vi "PH_ImageOperator.Fill Factor.vi"(0 "i ref in":refnum<vi>, 5 "error in":errorcluster) -> (14 "i ref out":refnum<vi>, 19 "error out":errorcluster)   [LabVIEW 2014, in "PH_ImageOperator.lvlib"]
doc: "This VI calculates the Fill factor."
uses:
  PH_ImageOperator.lvlib
  <vilib>/vision/NI_Vision_Development_Module.lvlib
  PH_Basics/PH_Common/PH_Common.lvlib
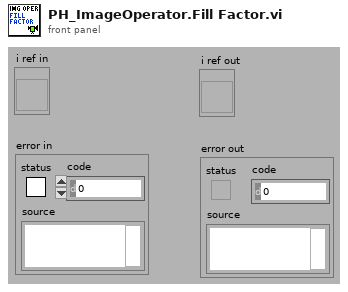
[diagram p1: front panel]
types:
  T1 = typedef "PH_ImageOperator.lvlib/PH_ImageOperator.i attribute.ctl" = cluster{"GUI Refs":cluster{"Delete":refnum<vi>, "Calibration status":refnum<vi>, "BI subtracted":refnum<vi>, "calc Energy":refnum<vi>, "Energy: expected value":refnum<vi>, "Energy: Tolerance":refnum<vi>, "Energy calculated":refnum<vi>, "Energy":refnum<vi>, "calc Beam Anal":refnum<vi>, "Maj Diam 1/esquare":refnum<vi>, "Min Diam 1/esquare":refnum<vi>, "Azi Angle":refnum<vi>, "Min/Maj Diam esquare":refnum<vi>, "Beam analysed":refnum<vi>, "CoG - x":refnum<vi>, "CoG - y":refnum<vi>, "BA: Method":refnum<vi>, "BA: Steps":refnum<vi>, "BA: Factor":refnum<vi>, "calc Traces":refnum<vi>, "Traces: Fit Gauss":refnum<vi>, "Traces calculated":refnum<vi>, "Maj FWHM":refnum<vi>, "Min FWHM":refnum<vi>, "Major Trace":refnum<vi>, "Minor Trace":refnum<vi>, "Maj Fit Order":refnum<vi>, "Min Fit Order":refnum<vi>, "Position calculated":refnum<vi>, "Position":refnum<vi>, "Type":refnum<vi>, "Center":refnum<vi>, "exp - X":refnum<vi>, "exp - Y":refnum<vi>, "Tolerance":refnum<vi>, "f":refnum<vi>, "M":refnum<vi>, "D":refnum<vi>, "q":refnum<vi>, "Dummy Method":refnum<vi>, "Dummy Type":refnum<vi>, "Global On":refnum<vi>, "Traces: No offset":refnum<vi>, "Maj 99%":refnum<vi>, "Min 99%":refnum<vi>, "GUI FF Image":refnum<vi>, "calc Fill Factor":refnum<vi>, "FF calculated":refnum<vi>, "Fill Factor: Filter?":refnum<vi>, "FF: Damage Threshold":refnum<vi>, "FF: Threshold":refnum<vi>, "FF: max allow. Energy":refnum<vi>, "FF: Fillfactor":refnum<vi>, "Calibration data":refnum<vi>}, "List of GUIs":string[], "Calibration":cluster{"Status":T2, "Calibration data":T3, "Calibration Data File":path}, "Final Image":cluster{"BI Subtraction Failure":bool}, "Energy":cluster{"on":bool, "expected value [mJ]":dbl, "Tolerance [%]":dbl, "State":T2, "Energy [mJ]":dbl, "Unit":string, "calculated @":timestamp}, "Beam Analysis":cluster{"on":bool, "Data":T4, "Method":bool, "Steps":i32, "Factor":i32, "ROI":cluster{"Left":i32, "Top":i32, "Right":i32, "Bottom":i32}, "analysed @":timestamp}, "Trace Analysis":cluster{"on":bool, "Fit on":bool, "Maj FWHM":dbl, "Min FWHM":dbl, "Maj Fit Order":i32, "Min Fit Order":i32, "No Offset":bool, "Maj 99%":dbl, "Min 99%":dbl, "Traces":cluster{"XScaleName":string, "Y Scale Minimum":sgl, "Y Scale Maximum":sgl, "X Scale Minimum":sgl, "X Scale Maximum":sgl, "Traces":cluster{"Index":sgl[], "Trace":dbl[]}[]}[], "analysed @":timestamp}, "Position Analysis":cluster{"on":bool, "exp - X":i32, "exp - Y":i32, "focal length [mm]":dbl, "Magnification":dbl, "Delta":dbl, "Theta":dbl, "Tolerance":dbl, "Type":bool, "analysed @":timestamp}, "Fill Factor":cluster{"on":bool, "Filter on?":bool, "Threshold":dbl, "Damage Threshold [J/cm²]":dbl, "Fillfactor":dbl, "Max. allowed Energy [J]":dbl, "calculated @":timestamp}, "Statistician Service ID":i32, "Images":cluster{"Background":T5, "OP":T5, "GUI":T5, "BA: ROI":T5, "Trace: Turn":T5, "FF: Main":T5, "FF: Help":T5, "PSDB: BG":T5, "PSDB: OP":T5, "PSDB: FF":T5}}
  T2 = typedef "PH_StatusHandler.lvlib/PH_StatusHandler.Status.ctl" = i16
  T3 = typedef "PH_ImageCalibrator.lvlib/PH_ImageCalibrator.Calibration Data.ctl" = cluster{"Date":string, "Time":string, "Cam Settings":cluster{"Cam ID":string, "Gain":dbl, "Brightness":dbl, "Shutter":dbl, "Cam Error":bool, "Mode":i32}, "Background Image":cluster{"Image":dbl[][], "Image Error":bool}, "Linear Calibration":cluster{"Calibration Factor":dbl, "not mm or mrad":bool}, "Energy Calibration":cluster{"Calibration Factor":dbl, "no mJ":bool}}
  T4 = typedef "PH_ImageOperator.lvlib/PH_ImageOperator.Beam Analysis Data.ctl" = cluster{"CoG-x":sgl, "CoG-y":sgl, "Maj Dim":dbl, "Min Dim":dbl, "Ellipticity":dbl, "Azimuth Angle [rad]":dbl, "Azi Angle rel to Maj?":bool}
  T5 = typedef "IMAQ Image.ctl" = refnum<image>
  T6 = typedef "Image Type" = u32
  T7 = cluster{"histogram":u32[], "Minimal Value":sgl, "Maximal Value":sgl, "Starting Value":sgl, "Interval Width":sgl, "Mean Value":sgl, "Standard  Variation":sgl, "Area (pixels)":i32}
  T8 = typedef "ROI Descriptor" = cluster{"Global Rectangle":i32[], "Contours":cluster{"ID":enum32{"External", "Internal"}, "Type":u32, "Coordinates":i32[]}[]}
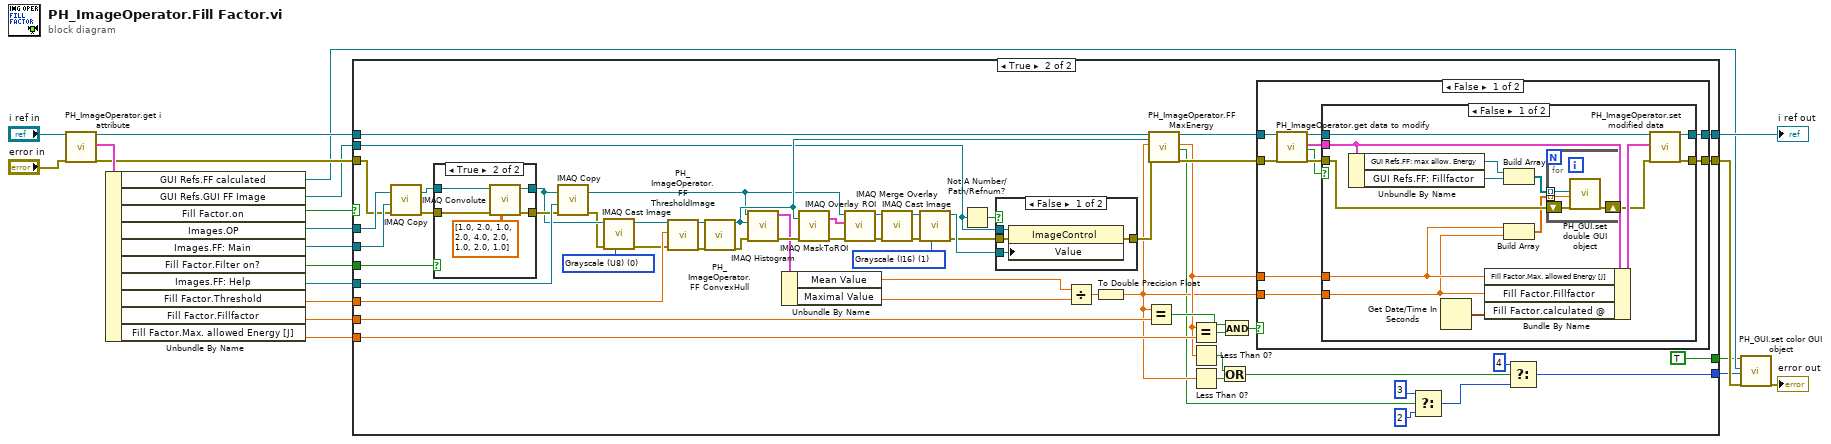
[diagram p0: block diagram]
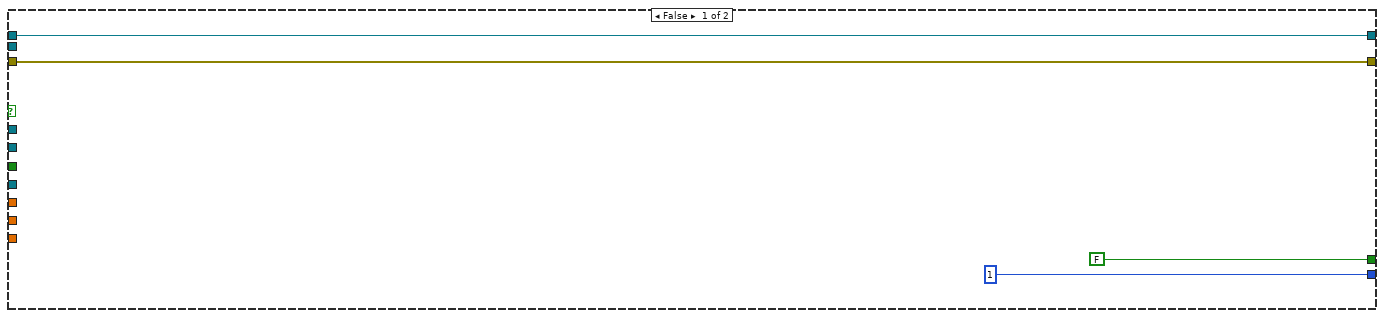
[diagram p2: hidden frame]
diagram:
  n1 = call "PH_ImageOperator.get i attribute.vi"("i ref in"="i ref in", "error in (no error)"="error in") -> ("i ref out"=w19:refnum<vi>, "i attribute"=w16:T1, "error out"=w15:errorcluster)  [unwired: 15 in]
  n2 = Unbundle By Name(w16) -> ("GUI Refs.FF calculated"=w8:refnum<vi>, "GUI Refs.GUI FF Image"=w9:refnum<vi>, "Fill Factor.on"=w17:bool, "Images.OP"=w3:T5, "Images.FF: Main"=w2:T5, "Fill Factor.Filter on?"=w10:bool, "Images.FF: Help"=w1:T5, "Fill Factor.Threshold"=w13:dbl, "Fill Factor.Fillfactor"=w11:dbl, "Fill Factor.Max. allowed Energy [J]"=w12:dbl)
  n3 = case shown="True" w17 {
    tunnel: [w23 w82] -> w6
    tunnel: [w24 w81] -> w14
    tunnel: w15 -> [w23 w63]
    tunnel: w19 -> [w24 w59]
    tunnel: w3 -> [_ w79]
    tunnel: w2 -> [_ w78]
    tunnel: w12 -> [_ w80]
    tunnel: w1 -> [_ w76]
    tunnel: w13 -> [_ w74]
    tunnel: w11 -> [_ w57]
    tunnel: w10 -> [_ w53]
    tunnel: w9 -> [_ w25]
    tunnel: [1 ("State") w34] -> w5
    tunnel: [FALSE TRUE] -> w4
    frame False {
    }
    frame True {
      w31 = T6 1 items=["Grayscale (U8)", "Grayscale (I16)", "Grayscale (SGL)", "Complex (CSG)", "RGB (U32)", "HSL (U32)", "RGB (U64)", "Grayscale (U16)"] ("Image Type")
      w46 = T6 0 items=["Grayscale (U8)", "Grayscale (I16)", "Grayscale (SGL)", "Complex (CSG)", "RGB (U32)", "HSL (U32)", "RGB (U64)"] ("Image Type")
      n4 = call "IMAQ Copy"("error in (no error)"=w63, "Image Dst"=w78, "Image Src"=w79) -> ("error out"=w77:errorcluster, "Image Dst Out"=w75:T5)  [unwired: 3 in]
      n5 = case shown="True" w53 {
        tunnel: [w89 w93] -> w44
        tunnel: w75 -> [w89 w92]
        tunnel: [w88 w91] -> w71
        tunnel: w77 -> [w88 w90]
        frame False {
        }
        frame True {
          n6 = call "IMAQ Convolute"("Kernel"=sgl[][] [[1.0, 2.0, 1.0], [2.0, 4.0, 2.0], [1.0, 2.0, 1.0]], "error in (no error)"=w90, "Image Src"=w92) -> ("error out"=w91:errorcluster, "Image Dst Out"=w93:T5)  [unwired: 7 in]
        }
      }
      n7 = call "IMAQ Copy"("error in (no error)"=w71, "Image Dst"=w76, "Image Src"=w44) -> ("error out"=w43:errorcluster, "Image Dst Out"=w52:T5)  [unwired: 3 in]
      n8 = call "IMAQ Cast Image"("Image Type"=w46, "error in (no error)"=w43, "Image Src"=w44) -> ("error out"=w42:errorcluster, "Image Dst Out"=w45:T5)  [unwired: 7 in]
      n9 = call "PH_ImageOperator.FF ThresholdImage.vi"("Image"=w45, "threshold"=w74, "error in (no error)"=w42) -> ("Image Dst Out"=w72:T5, "error out"=w73:errorcluster)  [unwired: 15 in]
      n10 = call "PH_ImageOperator.FF ConvexHull.vi"("Image Src"=w72, "error in (no error)"=w73) -> ("Image Dst Out"=w60:T5, "error out"=w67:errorcluster)  [unwired: 16 in]
      n11 = call "IMAQ Histogram"("error in (no error)"=w67, "Image Mask"=w60, "Image"=w52) -> ("error out"=w69:errorcluster, "Histogram Report"=w64:T7)  [unwired: 7 in]
      n12 = Unbundle By Name(w64) -> ("Mean Value"=w66:sgl, "Maximal Value"=w65:sgl)
      n13 = call "IMAQ MaskToROI"("Image"=w60, "error in (no error)"=w69) -> ("ROI Descriptor"=w70:T8, "error out"=w68:errorcluster)  [unwired: 5 in, 1 out]
      n14 = call "IMAQ Overlay ROI"("error in (no error)"=w68, "ROI Descriptor"=w70, "Image"=w52) -> ("error out"=w26:errorcluster, "Image Out"=w29:T5)  [unwired: 7 in]
      n15 = call "IMAQ Merge Overlay"("error in (no error)"=w26, "Image Src"=w29) -> ("error out"=w28:errorcluster, "Image Dst Out"=w32:T5)  [unwired: 8 in]
      n16 = call "IMAQ Cast Image"("Image Type"=w31, "error in (no error)"=w28, "Image Src"=w32) -> ("error out"=w27:errorcluster, "Image Dst Out"=w30:T5)  [unwired: 7 in]
      n17 = Not A Number/Path/Refnum?(number/path/refnum=w25) -> (NaN/Path/Refnum?=w50:bool)
      n18 = case shown="False" w50 {
        tunnel: w27 -> [w86 w87]
        tunnel: [w85 w87] -> w51
        tunnel: w25 -> [w84 _]
        tunnel: w30 -> [w83 _]
        frame False {
          n19 = property class="ImageControl"(reference=w84, error in=w86, "Value"=w83) -> (error out=w85:errorcluster)  [unwired: 1 out]
        }
        frame True {
        }
      }
      n20 = Divide(x=w66, y=w65) -> (x/y=w62:sgl)
      n21 = To Double Precision Float(number=w62) -> (double precision float=w40:dbl)
      n22 = Equal?(x=w40, y=w57) -> (x = y?=w56:bool)
      n23 = call "PH_ImageOperator.FF MaxEnergy.vi"("i ref in"=w59, "Image"=w60, "Fill Factor"=w40, "error in (no error)"=w51) -> ("i ref out"=w58:refnum<vi>, "Max. allowed energy (J)"=w41:dbl, "Error calculating the Energy?"=w33:bool, "error out"=w61:errorcluster)  [unwired: 12 in]
      n24 = Equal?(x=w41, y=w80) -> (x = y?=w55:bool)
      n25 = Less Than 0?(x=w41) -> (x < 0?=w39:bool)
      n26 = Less Than 0?(x=w40) -> (x < 0?=w38:bool)
      n27 = Or(x=w39, y=w38) -> (x .or. y?=w37:bool)
      n28 = And(x=w56, y=w55) -> (x .and. y?=w54:bool)
      n29 = case shown="False" w54 {
        tunnel: [w104 w125] -> w82
        tunnel: [w103 w126] -> w81
        tunnel: w58 -> [w98 w126]
        tunnel: w61 -> [w97 w125]
        tunnel: w40 -> [w96 _]
        tunnel: w41 -> [w95 _]
        frame False {
          n30 = call "PH_ImageOperator.get data to modify.vi"("i ref in"=w98, "error in (no error)"=w97) -> ("i ref out"=w102:refnum<vi>, "i attribute"=w99:T1, "timed out"=w100:bool, "error out"=w101:errorcluster)  [unwired: 14 in]
          n31 = case shown="False" w100 {
            tunnel: [w116 w123] -> w104
            tunnel: [w115 w124] -> w103
            tunnel: w102 -> [w118 w124]
            tunnel: w101 -> [w113 w123]
            tunnel: w99 -> [w114 _]
            tunnel: w96 -> [w110 _]
            tunnel: w95 -> [w111 _]
            frame False {
              n32 = Unbundle By Name(w114) -> ("GUI Refs.FF: max allow. Energy"=w108:refnum<vi>, "GUI Refs.FF: Fillfactor"=w107:refnum<vi>)
              n33 = Get Date/Time In Seconds() -> (seconds since 1Jan1904=w105:timestamp)
              n34 = Bundle By Name(cluster=w114, "Fill Factor.Max. allowed Energy [J]"=w111, "Fill Factor.Fillfactor"=w110, "Fill Factor.calculated @"=w105) -> (w117:T1)
              n35 = Build Array(w108, w107) -> (w106:refnum<vi>[])
              n36 = Build Array(w111, w110) -> (w109:dbl[])
              n37 = for {
                tunnel: w109 -> [w120] mode=indexing
                tunnel: w106 -> [w119] mode=indexing
                shift-right: [w121] -> w112
                shift-left: w113 -> [w122]
                n38 = call "PH_GUI.set double GUI object.vi"("GUI object Ref"=w119, "value"=w120, "error in (no error)"=w122) -> ("error out"=w121:errorcluster)  [unwired: 16 in]
              }
              n39 = call "PH_ImageOperator.set modified data.vi"("i ref in"=w118, "i attribute"=w117, "error in (no error)"=w112) -> ("i ref out"=w115:refnum<vi>, "error out"=w116:errorcluster)  [unwired: 15 in]
            }
            frame True {
            }
          }
        }
        frame True {
        }
      }
      n40 = Select(t=3 ("State"), s=w33, f=2 ("State")) -> (s? t:f=w35:i32)
      n41 = Select(t=4, s=w37, f=w35) -> (s? t:f=w34:i32)
    }
  }
  "i ref out" <- w14
  n42 = call "PH_GUI.set color GUI object.vi"("Visible? (true)"=w4, "GUI object Ref"=w8, "State"=w5, "error in (no error)"=w6) -> ("error out"=→"error out":errorcluster)  [unwired: 15 in]
